vi "trajectory of ball.vi"() -> ()   [LabVIEW 2014]
panel:
  out "y":dbl
  out "x":dbl
  out "radius":dbl
  out "Boolean":bool
  out "initial energy":dbl
  out "V2":dbl
  in  "percentage threshold of energy remained":dbl
  in  "percentage of energy loss":dbl
  in  "initial angel":dbl
  in  "initial velocity":dbl
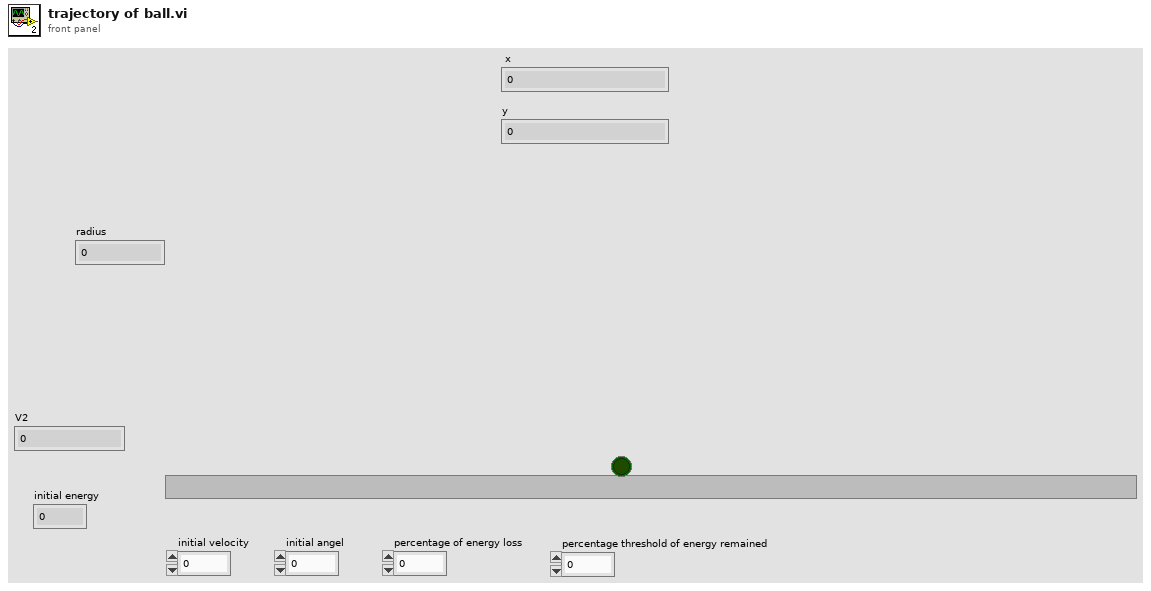
[diagram p1: front panel]
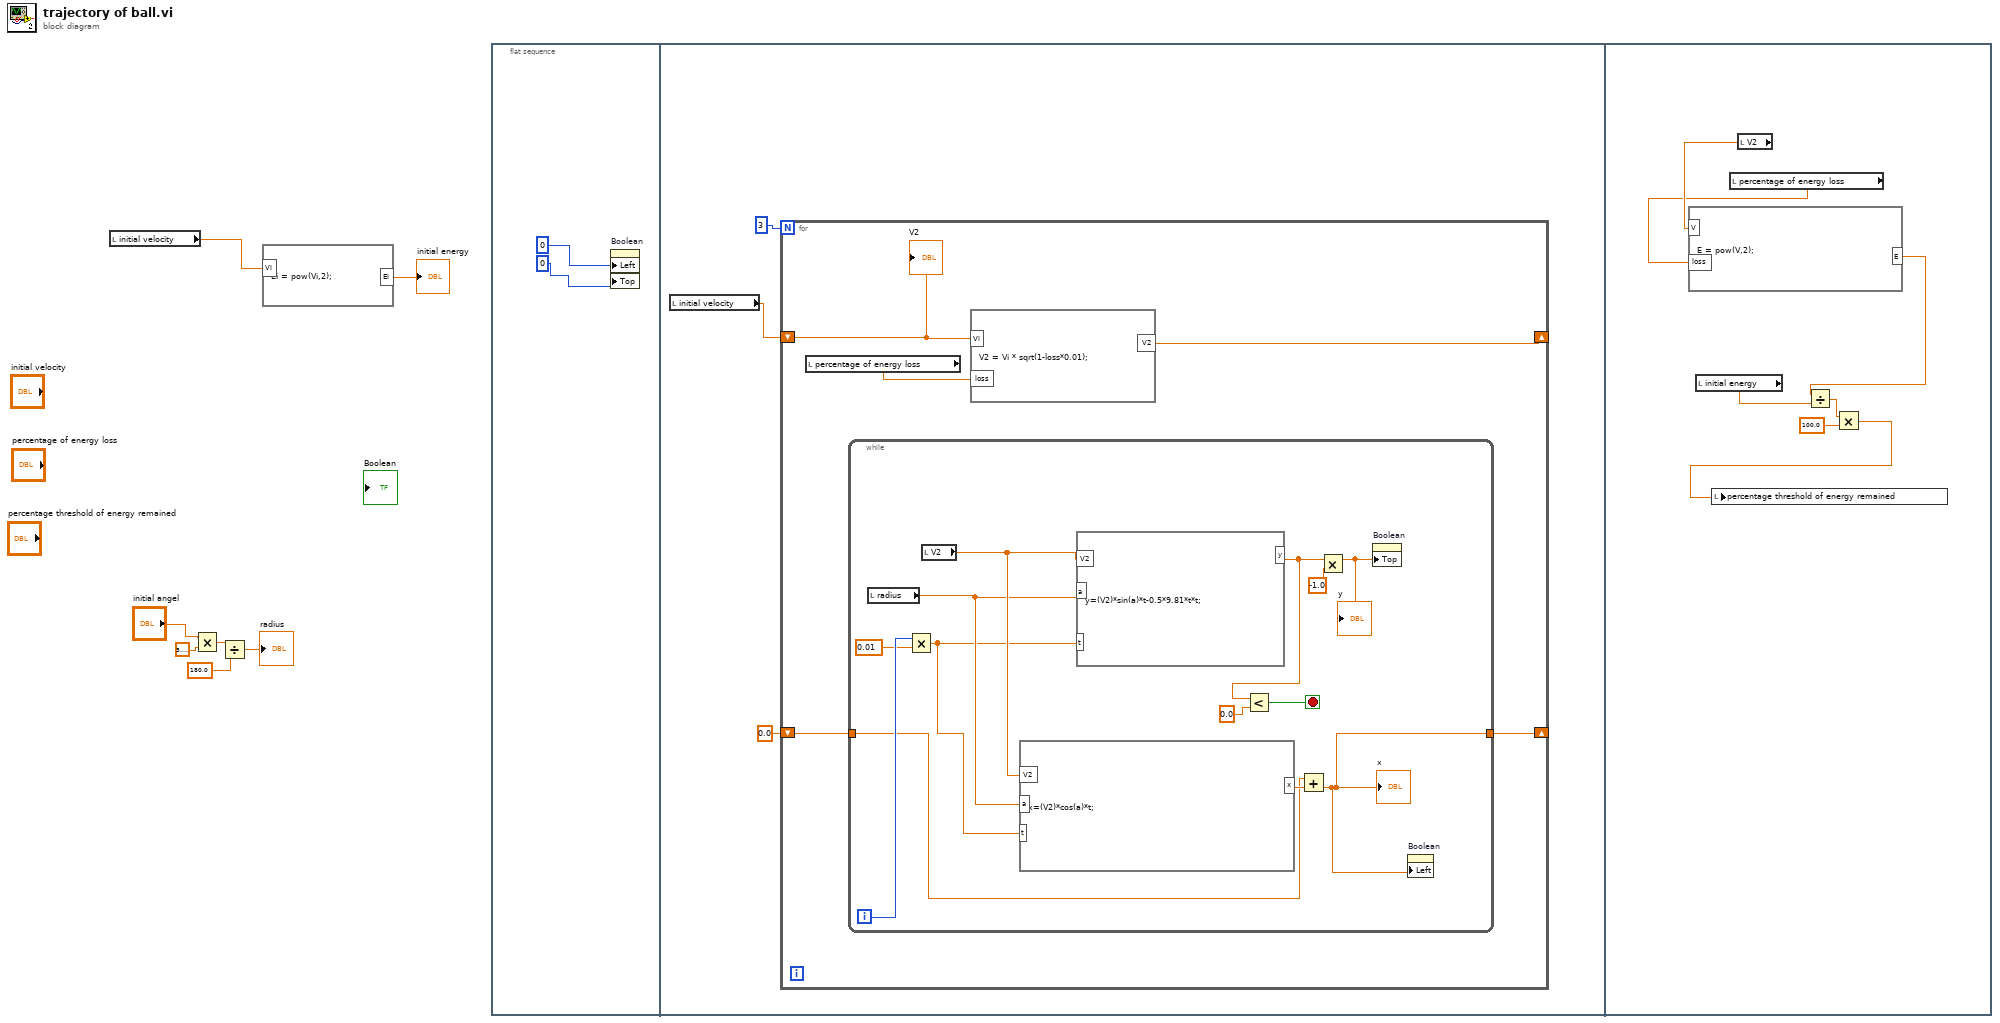
[diagram p0: block diagram]
diagram:
  n1 = local read "initial velocity"() -> (w6:dbl)
  n2 = Multiply(x="initial angel", y=3.141592653589793) -> (x*y=w3:dbl)
  n3 = Divide(x=w3, y=180.0) -> (x/y=→"radius":dbl)
  n4 = formula code="Ei = pow(Vi,2);"("Vi"=w6) -> ("Ei"=→"initial energy":dbl)
  n5 = flat-sequence {
    frame #0 {
      n6 = property on="Boolean" class="Bool (strict)"("Left"=0 ("Position:Top"), "Top"=0 ("Position:Left")) -> ()  [unwired: 2 in, 2 out]
    }
    frame #1 {
      n7 = local read "initial velocity"() -> (w12:dbl)
      n8 = for {
        N: 3 -> [_]
        shift-right: [w16] -> _
        shift-left: w12 -> [w15]
        shift-right: [w14] -> _
        shift-left: 0.0 -> [w13]
        n9 = local read "percentage of energy loss"() -> (w17:dbl)
        n10 = while {
          tunnel: w13 -> [w18]
          tunnel: [w19] -> w14
          i -> [w27]
          stop <- w30 stop-if-true
          n11 = local read "radius"() -> (w24:dbl)
          n12 = Multiply(x=w27, y=0.01) -> (x*y=w20:dbl)
          n13 = local read "V2"() -> (w29:dbl)
          n14 = formula code="x=(V2)*cos(a)*t;"("V2"=w29, "t"=w20, "a"=w24) -> ("x"=w21:dbl)
          n15 = formula code="y=(V2)*sin(a)*t-0.5*9.81*t*t;"("V2"=w29, "a"=w24, "t"=w20) -> ("y"=w25:dbl)
          n16 = Less?(x=w25, y=0.0) -> (x < y?=w30:bool)
          n17 = Add(x=w18, y=w21) -> (x+y=w19:dbl)
          "x" <- w19
          n18 = Multiply(x=w25, y=-1.0) -> (x*y=w23:dbl)
          "y" <- w23
          n19 = property on="Boolean" class="Bool (strict)"("Top"=w23) -> ()  [unwired: 2 in, 2 out]
          n20 = property on="Boolean" class="Bool (strict)"("Left"=w19) -> ()  [unwired: 2 in, 2 out]
        }
        n21 = formula code="V2 = Vi * sqrt(1-loss*0.01);"("Vi"=w15, "loss"=w17) -> ("V2"=w16:dbl)
        "V2" <- w15
      }
    }
    frame #2 {
      n22 = local read "initial energy"() -> (w31:dbl)
      n23 = local read "percentage of energy loss"() -> (w32:dbl)
      n24 = local read "V2"() -> (w34:dbl)
      n25 = formula code="E = pow(V,2);"("V"=w34, "loss"=w32) -> ("E"=w33:dbl)
      n26 = Divide(x=w33, y=w31) -> (x/y=w37:dbl)
      n27 = Multiply(x=w37, y=100.0) -> (x*y=w35:dbl)
      n28 = local write "percentage threshold of energy remained"(w35) -> ()
    }
  }
